vi "管理机.vi"() -> ()   [LabVIEW 2015]
uses:
  <vilib>/Modbus/master/Modbus Master.lvclass
  Global control/global-1.vi
  <userlib>/QMH/Message Queue/Support/Enqueue Message (Single).vi
  <vilib>/Modbus/master/Create Master Instance (Serial).vi
  <userlib>/QMH/Message Queue/Message Queue.lvlib
panel:
  in  "HostThread":variant
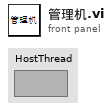
[diagram p1: front panel]
types:
  T1 = cluster{"Controls":cluster{"Exit":refnum<vi>}, "Thread":cluster{"ThisQ":string, "ThisVI":refnum<vi>, "HostQ":string, "HostRef":refnum<vi>, "SlavesQ":string[], "SlavesRef":refnum<vi>[]}, "Data":cluster{"Replace":bool}, "User":cluster{"Name":string}, "Modbus master ":refnum<class "Modbus Master.lvclass">}
  T2 = cluster{bool, bool, bool, bool, bool, bool, bool, bool, bool, bool, bool, bool, bool, bool, bool, bool}
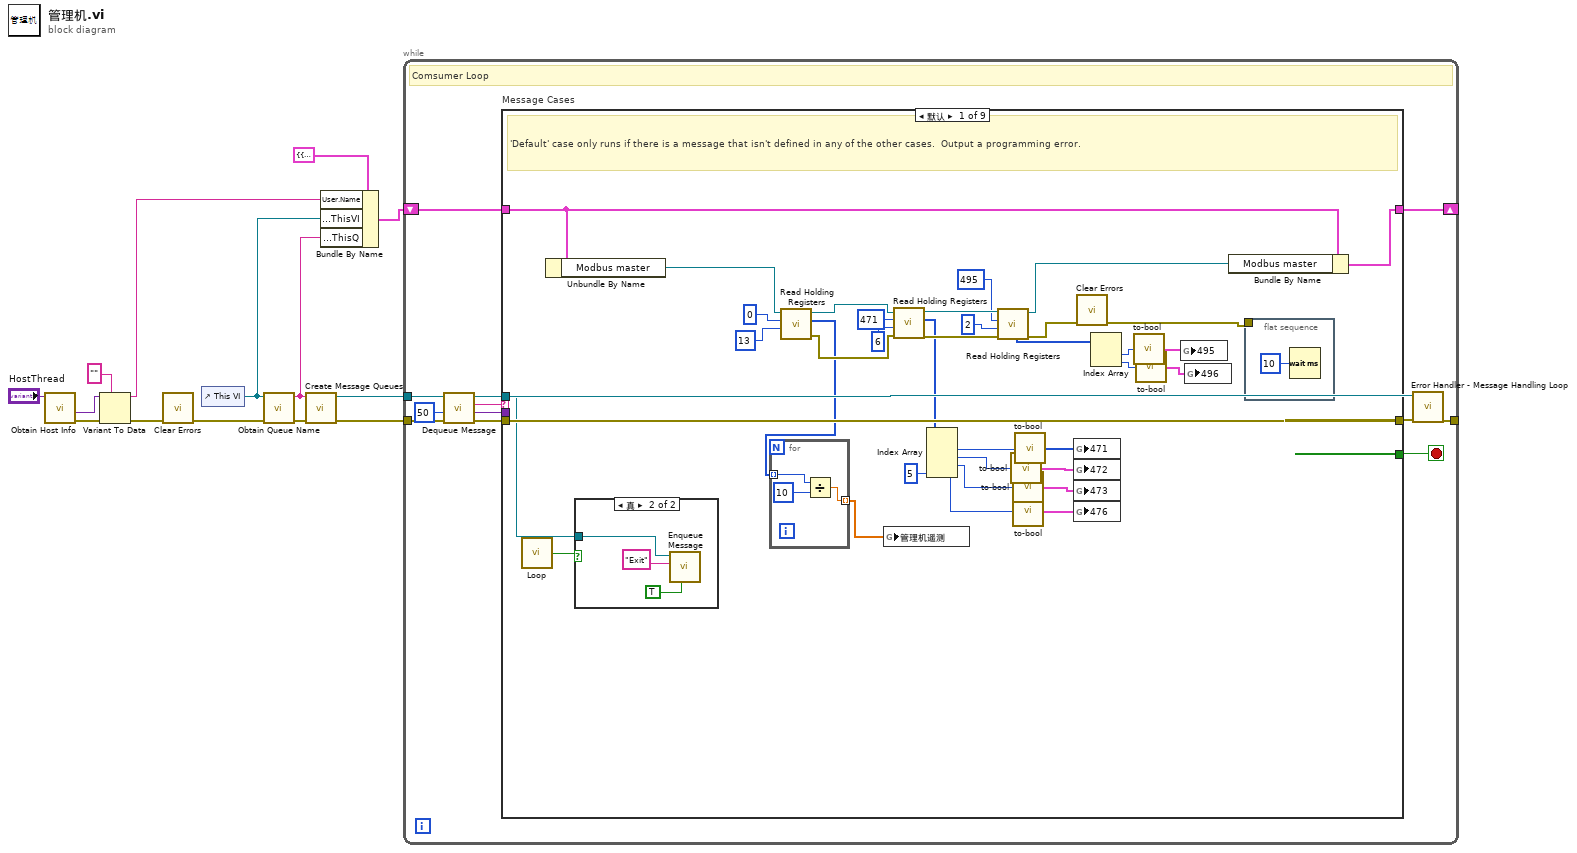
[diagram p0: block diagram]
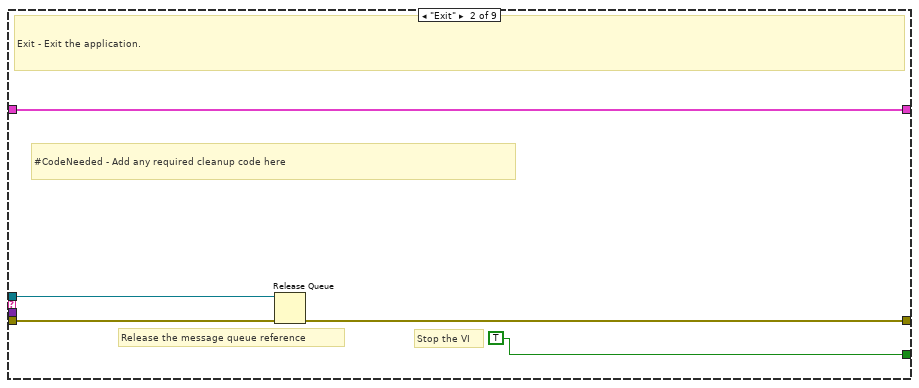
[diagram p3: hidden frame]
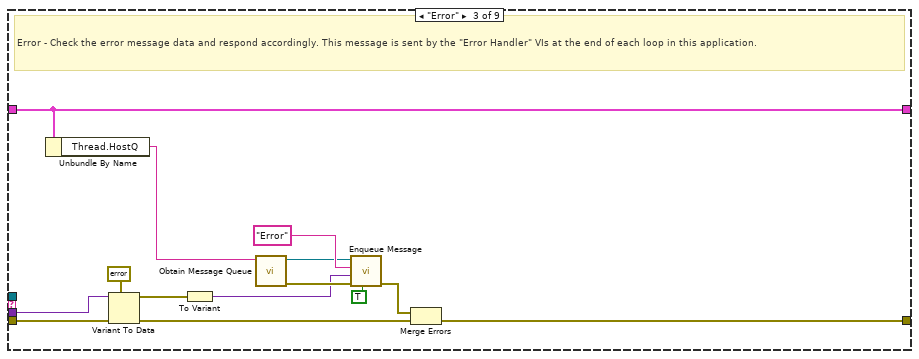
[diagram p4: hidden frame]
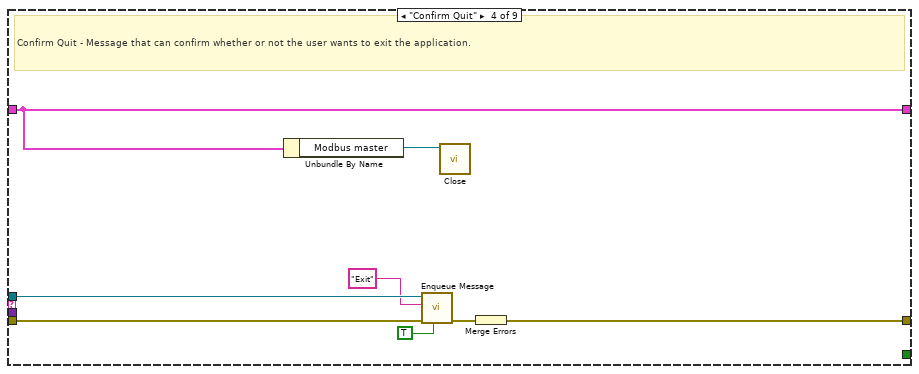
[diagram p5: hidden frame]
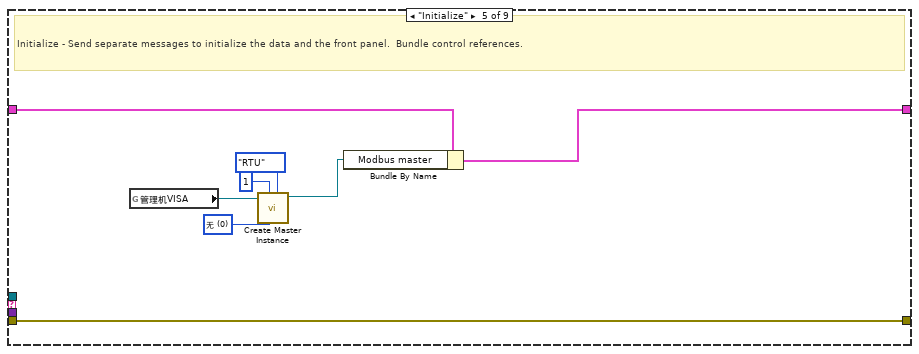
[diagram p6: hidden frame]
diagram:
  n1 = call <userlib>:"Obtain Host Info.vi"("HostThread"="HostThread") -> ("error out"=w6:errorcluster, "Data"=w5:variant)  [unwired: 7 in, 2 out]
  n2 = Variant To Data(error in=w6, type="", Variant=w5) -> (data=w1:string, error out=w3:errorcluster)
  n3 = call <vilib>:"Clear Errors.vi"("error in (no error)"=w3) -> ("error out"=w2:errorcluster)  [unwired: 5 in, 1 out]
  n4 = control-ref of="This VI"() -> (w10:refnum<vi>)
  n5 = call <userlib>:"Obtain Queue Name.vi"("error in (no error)"=w2, "VI Refnum"=w10) -> ("error out"=w13:errorcluster, "ViName"=w9:string)  [unwired: 8 in]
  n6 = call <userlib>:"Create Message Queues.vi"("error in (no error)"=w13, "name (unnamed)"=w9) -> ("error out"=w14:errorcluster, "QueueHandler"=w7:refnum<queue>)  [unwired: 8 in]
  n7 = Bundle By Name(cluster=T1 {"Controls"={"Exit"=refnum}, "Thread"={"ThisQ"="", "ThisVI"=refnum, "HostQ"="", "HostRef"=refnum, "SlavesQ"=[], "SlavesRef"=[]}, "Data"={"Replace"=FALSE}, "User"={"Name"=""}, "Modbus master "=refnum} ("Data Cluster"), "User.Name"=w1, "Thread.ThisVI"=w10, "Thread.ThisQ"=w9) -> (w11:T1)
  n8 = while {
    tunnel: w7 -> [w19]
    shift-right: [w25] -> _
    shift-left: w11 -> [w26]
    tunnel: w14 -> [w23]
    tunnel: [w17] -> _
    stop <- w24 stop-if-true
    # "Comsumer Loop"
    n9 = call <userlib>:"Dequeue Message.vi"("error in (no error)"=w23, "timeout in ms (-1)"=50, "Message Queue"=w19) -> ("error out"=w22:errorcluster, "Message Data"=w20:variant, "Message"=w21:string, "dup Message Queue"=w18:refnum<queue>)  [unwired: 5 in]
    n10 = case "Message Cases" shown="默认" w21 {
      tunnel: w18 -> [w44 w74 _ w93 _ _ _ _ _]
      tunnel: w22 -> [w62 w71 w88 w96 w104 w106 w108 w109 w112]
      tunnel: [w62 w70 w83 w95 w104 w106 w108 w109 w112] -> w16
      tunnel: w26 -> [w59 w73 w80 w90 w98 w105 w107 w110 w111]
      tunnel: [w58 w73 w80 w90 w97 w105 w107 w110 w111] -> w25
      tunnel: [_ TRUE _ _ _ _ _ _ _] -> w24
      tunnel: w20 -> [_ _ w87 _ _ _ _ _ _]
      frame Default {
        # "'Default' case only runs if there is a message that isn't defined in any of the other cases.  Output a programming error."
        n11 = call "Loop.vi"() -> ("Loop Out"=w45:bool)  [unwired: 5 in]
        n12 = Unbundle By Name(w59) -> ("Modbus master"=w32:refnum<class "Modbus Master.lvclass">)
        n13 = case shown="真" w45 {
          tunnel: w44 -> [_ w67]
          frame False {
          }
          frame True {
            n14 = call-poly <userlib>:"Enqueue Message.vi"("Priority Message? (F)"=TRUE, "Message"="Exit", "Message Queue"=w67) -> ()  [unwired: 7 in, 2 out]
          }
        }
        n15 = call-dynamic "Read Holding Registers.vi"("number of holding registers"=u16 13, "starting address"=u16 0, "Modbus master in"=w32) -> ("error out"=w52:errorcluster, "register values"=w35:u16[], "Modbus master out"=w57:refnum<class "Modbus Master.lvclass">)  [unwired: 6 in]
        n16 = for {
          tunnel: w35 -> [w66] mode=indexing
          tunnel: [w64] -> w34 mode=indexing
          n17 = Divide(x=w66, y=u16 10) -> (x/y=w64:dbl)
        }
        n18 = global write "global-1.vi" "管理机遥测"(w34) -> ()
        n19 = call-dynamic "Read Holding Registers.vi"("error in (no error)"=w52, "number of holding registers"=u16 6, "starting address"=u16 471, "Modbus master in"=w57) -> ("error out"=w53:errorcluster, "register values"=w47:u16[], "Modbus master out"=w54:refnum<class "Modbus Master.lvclass">)  [unwired: 5 in]
        n20 = Index Array(array=w47, index #4=5 ("索引")) -> (element #1=w46:u16, element #2=w42:u16, element #3=w39:u16, element #4=w37:u16)  [unwired: 3 in]
        n21 = call-dynamic "Read Holding Registers.vi"("error in (no error)"=w53, "number of holding registers"=u16 2, "starting address"=u16 495, "Modbus master in"=w54) -> ("error out"=w51:errorcluster, "register values"=w33:u16[], "Modbus master out"=w50:refnum<class "Modbus Master.lvclass">)  [unwired: 5 in]
        n22 = call "to-bool.vi"("register"=w42) -> ("簇"=w41:T2)
        n23 = call "to-bool.vi"("register"=w39) -> ("簇"=w40:T2)
        n24 = call "to-bool.vi"("register"=w37) -> ("簇"=w36:T2)
        n25 = call "to-bool.vi"("register"=w46) -> ("簇"=w43:T2)
        n26 = global write "global-1.vi" "471"(w43) -> ()
        n27 = global write "global-1.vi" "472"(w41) -> ()
        n28 = global write "global-1.vi" "473"(w40) -> ()
        n29 = global write "global-1.vi" "476"(w36) -> ()
        n30 = call <vilib>:"Clear Errors.vi"("error in (no error)"=w51) -> ("error out"=w27:errorcluster)  [unwired: 5 in, 1 out]
        n31 = Index Array(array=w33) -> (element #1=w31:u16, element #2=w29:u16)  [unwired: 2 in]
        n32 = call "to-bool.vi"("register"=w31) -> ("簇"=w30:T2)
        n33 = call "to-bool.vi"("register"=w29) -> ("簇"=w28:T2)
        n34 = global write "global-1.vi" "495"(w30) -> ()
        n35 = global write "global-1.vi" "496"(w28) -> ()
        n36 = Bundle By Name(cluster=w59, "Modbus master"=w50) -> (w58:T1)
        n37 = flat-sequence {
          tunnel: w27 -> [_]
          frame #0 {
            n38 = Wait (ms)(milliseconds to wait=u32 10 ("等待时间（毫秒）")) -> ()  [unwired: 1 out]
          }
        }
      }
      frame "Exit" {
        # "Stop the VI"
        # "Release the message queue reference"
        # "#CodeNeeded - Add any required cleanup code here"
        # "Exit - Exit the application."
        n39 = Release Queue(queue=w74, error in (no error)=w71) -> (error out=w70:errorcluster)  [unwired: 1 in, 2 out]
      }
      frame "Error" {
        # "Error - Check the error message data and respond accordingly. This message is sent by the \"Error Handler\" VIs at the end of each loop in this application."
        n40 = Unbundle By Name(w80) -> ("Thread.HostQ"=w79:string)
        n41 = Variant To Data(error in=w88, type=errorcluster {"status"=FALSE, "code"=0, "source"=""} ("error constant"), Variant=w87) -> (data=w76:errorcluster, error out=w85:errorcluster)
        n42 = To Variant(anything=w76) -> (Variant=w75:variant)
        n43 = call <userlib>:"Obtain Message Queue.vi"("name (unnamed)"=w79) -> ("error out"=w78:errorcluster, "Message Queue"=w77:refnum<queue>)  [unwired: 9 in]
        n44 = call-poly <userlib>:"Enqueue Message.vi"("Priority Message? (F)"=TRUE, "error in (no error)"=w78, "Message Data"=w75, "Message"="Error", "Message Queue"=w77) -> ("error out"=w84:errorcluster)  [unwired: 5 in, 1 out]
        n45 = Merge Errors(w84, w85) -> (w83:errorcluster)
      }
      frame "Confirm Quit" {
        # "Confirm Quit - Message that can confirm whether or not the user wants to exit the application."
        n46 = Unbundle By Name(w90) -> ("Modbus master"=w89:refnum<class "Modbus Master.lvclass">)
        n47 = call-poly <userlib>:"Enqueue Message.vi"("Priority Message? (F)"=TRUE, "error in (no error)"=w96, "Message"="Exit", "Message Queue"=w93) -> ("error out"=w94:errorcluster)  [unwired: 6 in, 1 out]
        n48 = call-dynamic "Close.vi"("Modbus master in"=w89) -> ()  [unwired: 10 in, 1 out]
        n49 = Merge Errors(w94) -> (w95:errorcluster)
      }
      frame "Initialize" {
        w103 = u16 0 items=["无", "奇", "偶"] ("parity (Even)")
        # "Initialize - Send separate messages to initialize the data and the front panel.  Bundle control references."
        n50 = global read "global-1.vi" "管理机VISA"() -> (w101:refnum<visa-resource-name>)
        n51 = call-poly <vilib>:"Create Master Instance.vi"("serial type"=enum16{"RTU", "ASCII"}."RTU", "parity (Even)"=w103, "unit ID"=u8 1, "VISA resource name"=w101) -> ("serial master instance"=w99:refnum<class "Modbus Master.lvclass">)  [unwired: 6 in, 1 out]
        n52 = Bundle By Name(cluster=w98, "Modbus master"=w99) -> (w97:T1)
      }
      frame "<-------UI-------->" {
      }
      frame "<------Core------>" {
      }
      frame "Core_InitializeRef" {
        # "Initialize control references. For there is not enough space to locate all the control references, separate the codes into 2 messages"
      }
      frame "<---Operation--->" {
      }
    }
    n53 = call <userlib>:"Error Handler - Message Handling Loop.vi"("error in (no error)"=w16, "Message Queue"=w18) -> ("dup error in"=w17:errorcluster)  [unwired: 8 in, 1 out]
  }
